vi "frontp_replace_hardware_caller_queue.vi"(8 "error in (no error)":errorcluster, 9 "Nested Actor's Enqueuer":refnum<class "Message Enqueuer.lvclass">, 10 "hardware":T1, 11 "front_panel in":refnum<class "front_panel.lvclass">) -> (0 "error out":errorcluster, 3 "front_panel out":refnum<class "front_panel.lvclass">)   [LabVIEW 2015, in "front_panel.lvclass"]
uses:
  front_panel.lvclass
  hardware_caller_queue_numbers.ctl
  <vilib>/ActorFramework/Message Enqueuer/Message Enqueuer.lvclass
  front_panel.lvclass/front_panel.ctl
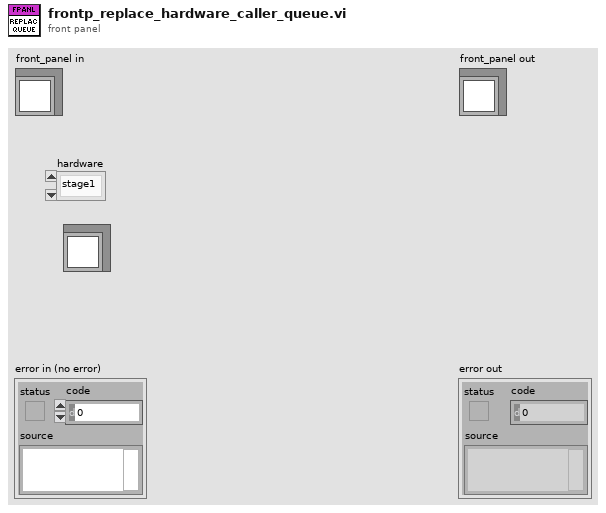
[diagram p1: front panel]
types:
  T1 = typedef "hardware_caller_queue_numbers.ctl" = enum16{"stage1", "stage2", "experiment", "detector"}
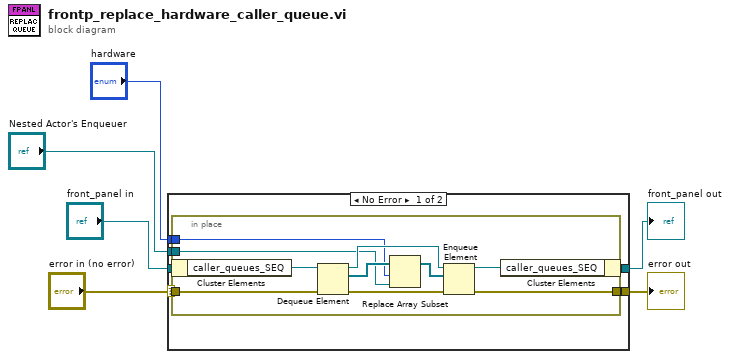
[diagram p0: block diagram]
diagram:
  n1 = case shown="No Error" "error in (no error)" {
    selector: "error in (no error)" -> [w11 w24]
    tunnel: [w9 w24] -> w5
    tunnel: [w8 w23] -> w3
    tunnel: "front_panel in" -> [w12 w23]
    tunnel: "hardware" -> [w10 _]
    tunnel: "Nested Actor's Enqueuer" -> [w7 _]
    frame No Error {
      n2 = in-place {
        in-place-border: w11 -> [w21]
        in-place-border: w10 -> [w15]
        in-place-border: [w17] -> w9
        in-place-border: w7 -> [w13]
        n3 = in-place-cluster #1(w12) -> ("caller_queues_SEQ"=w22:refnum<queue>)
        n4 = Dequeue Element(queue=w22, error in (no error)=w21) -> (queue out=w19:refnum<queue>, element=w16:refnum<class "Message Enqueuer.lvclass">[], error out=w20:errorcluster)  [unwired: 1 in, 1 out]
        n5 = Replace Array Subset(array=w16, new element=w13, index=w15) -> (w14:refnum<class "Message Enqueuer.lvclass">[])
        n6 = Enqueue Element(queue=w19, element=w14, error in (no error)=w20) -> (queue out=w18:refnum<queue>, error out=w17:errorcluster)  [unwired: 1 in, 1 out]
        n7 = in-place-cluster #1("caller_queues_SEQ"=w18) -> (w8:refnum<class "front_panel.lvclass">)
      }
    }
    frame Error {
    }
  }
  "error out" <- w5
  "front_panel out" <- w3
